vi "Rack-Config.vi"(8 "error in (no error)":errorcluster, 11 "Options":T1={"Input polling period (ms)"=2, "Logfile folder"=path "C:/Users/SiapasLab/Desktop/git/wheatley/test_log.txt"}) -> (0 "error out":errorcluster, 3 "Configuration":T2={"DigitalInput"={"Lines"=["6289/port1/line0", "6289/port1/line1", "6289/port1/line2", "6289/port1/line3", "6289/port1/line4", "6289/port1/line5", "6289/port1/line6", "6289/port1/line7"], "Refresh period (ms)"=0}, "DigitalOutput"={"Output Lines"=["6289/port0/line1", "6289/port0/line2", "6289/port0/line3", "6289/port0/line4", "6289/port0/line5", "6289/port0/line6", "6289/port0/line7"], "DO timestamp lines"=["6289/port0/line1", "6289/port0/line2", "6289/port0/line3", "6289/port0/line4", "6289/port0/line5", "6289/port0/line6", "6289/port0/line7"], "Timestamp lines"=[]}, "FileOutput"={"Logfile path"=path ""}, "AnalogOutput"={"Output Lines"=["6289/port0/line1", "6289/port0/line2", "6289/port0/line3", "6289/port0/line4", "6289/port0/line5", "6289/port0/line6", "6289/port0/line7"], "AO timestamp lines"=["6289/port0/line1", "6289/port0/line2", "6289/port0/line3", "6289/port0/line4", "6289/port0/line5", "6289/port0/line6", "6289/port0/line7"]}, "DataSocketOutput"={"DataSocket URL"=""}})   [LabVIEW 2015]
doc: "Creates an appropriate configuration cluster for use in Rack-Start.vi\n\nOptions are specified in this VI's front panel, but can be overwritten by the calling VI (just use bundle by name).\n\nCall this after all devices are initialized, as it uses the port reservation system to find which lines to assign to each port driver."
uses:
  Typedefs/Rack driver configuration cluster.ctl
  Port drivers/DigitalInput-Configuration.ctl
  Port drivers/DigitalOutput-Configuration.ctl
  Port drivers/FileOutput-Configuration.ctl
  Port drivers/AnalogOutput-Configuration.ctl
  Port drivers/DataSocketOutput-Configuration.ctl
panel:
  # "Timestamp lines must be on an M-Series card (i.e. NOT the 6509)"
  # "Timestamp lines must be on same device as its corresponding DO line"
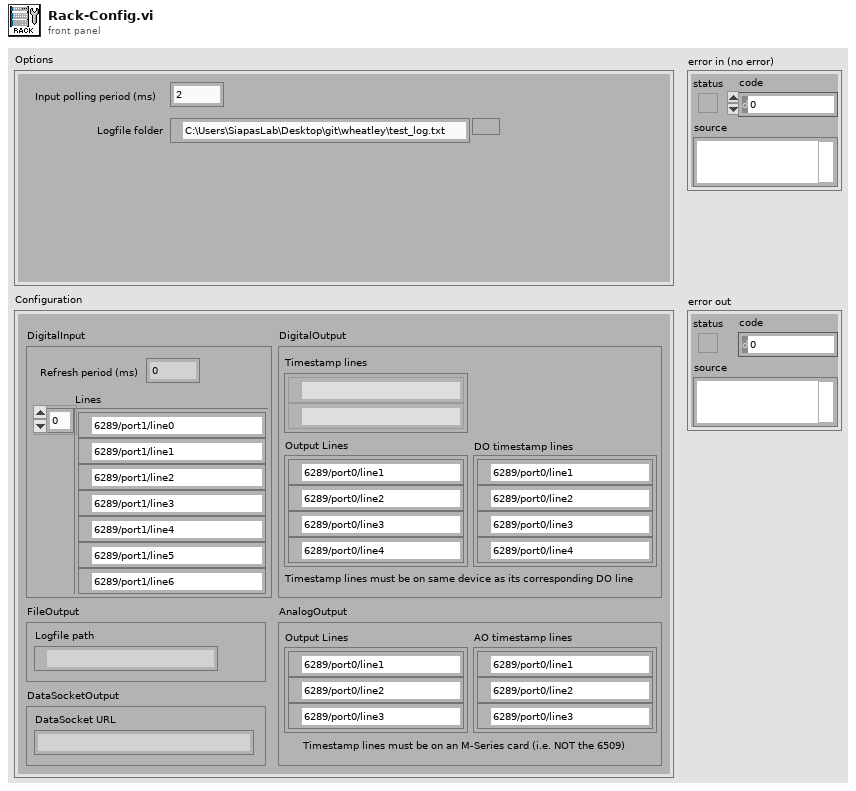
[diagram p1: front panel]
types:
  T1 = cluster{"Input polling period (ms)":u32, "Logfile folder":path}
  T2 = typedef "Rack driver configuration cluster.ctl" = cluster{"DigitalInput":T3, "DigitalOutput":T4, "FileOutput":T5, "AnalogOutput":T6, "DataSocketOutput":T7}
  T3 = typedef "DigitalInput-Configuration.ctl" = cluster{"Lines":tag[], "Refresh period (ms)":u32}
  T4 = typedef "DigitalOutput-Configuration.ctl" = cluster{"Output Lines":tag[], "DO timestamp lines":tag[], "Timestamp lines":tag[]}
  T5 = typedef "FileOutput-Configuration.ctl" = cluster{"Logfile path":path}
  T6 = typedef "AnalogOutput-Configuration.ctl" = cluster{"Output Lines":tag[], "AO timestamp lines":tag[]}
  T7 = typedef "DataSocketOutput-Configuration.ctl" = cluster{"DataSocket URL":string}
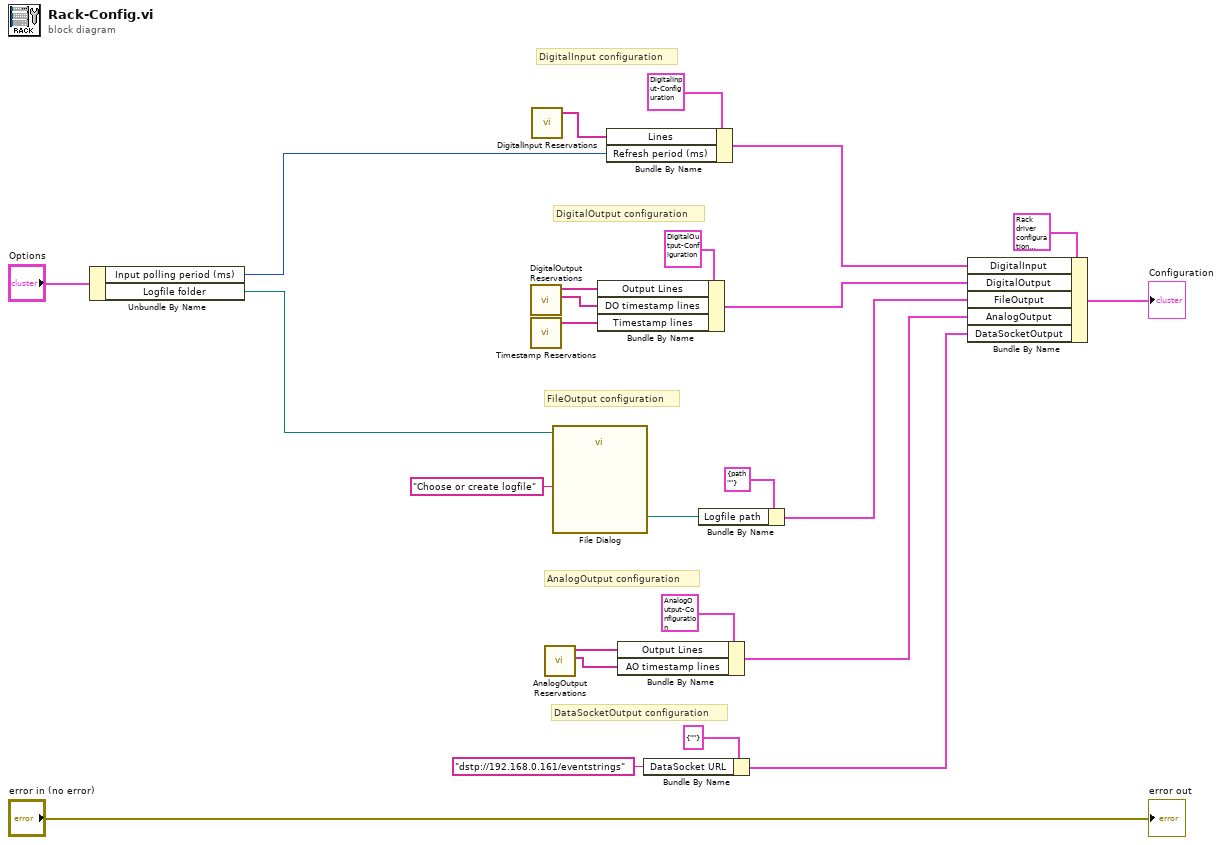
[diagram p0: block diagram]
diagram:
  # "DataSocketOutput configuration"
  # "AnalogOutput configuration"
  # "FileOutput configuration"
  # "DigitalOutput configuration"
  # "DigitalInput configuration"
  n1 = Unbundle By Name("Options") -> ("Input polling period (ms)"=w20:u32, "Logfile folder"=w14:path)
  n2 = call "DigitalOutput Reservations.vi"() -> ("DO timestamp lines"=w9:tag[], "DigitalOutput lines"=w17:tag[])  [unwired: 4 in, 2 out]
  n3 = call "Timestamp Reservations.vi"() -> ("DigitalOutput lines"=w8:tag[])  [unwired: 3 in, 2 out]
  n4 = call "DigitalInput Reservations.vi"() -> ("DigitalInput lines"=w19:tag[])  [unwired: 3 in, 2 out]
  n5 = call "AnalogOutput Reservations.vi"() -> ("AO timestamp lines"=w4:tag[], "AnalogOutput lines"=w5:tag[])  [unwired: 4 in, 2 out]
  n6 = call "File Dialog"("start path"=w14, "prompt"="Choose or create logfile") -> ("selected path"=w10:path)  [unwired: 10 in, 3 out]
  n7 = Bundle By Name(cluster=T4 {"Output Lines"=["6289/port0/line3", "6289/port0/line4", "6289/port0/line5", "6289/port0/line6", "6289/port0/line7"], "DO timestamp lines"=[], "Timestamp lines"=[]} ("DigitalOutput"), "Output Lines"=w17, "DO timestamp lines"=w9, "Timestamp lines"=w8) -> (w15:T4)
  n8 = Bundle By Name(cluster=T3 {"Lines"=["6289/port1/line0", "6289/port1/line1", "6289/port1/line2", "6289/port1/line3", "6289/port1/line4", "6289/port1/line5", "6289/port1/line6", "6289/port1/line7"], "Refresh period (ms)"=0} ("DigitalInput"), "Lines"=w19, "Refresh period (ms)"=w20) -> (w16:T3)
  n9 = Bundle By Name(cluster=T6 {"Output Lines"=["6289/port0/line1", "6289/port0/line2", "6289/port0/line3", "6289/port0/line4", "6289/port0/line5", "6289/port0/line6", "6289/port0/line7"], "AO timestamp lines"=["6289/port0/line1", "6289/port0/line2", "6289/port0/line3", "6289/port0/line4", "6289/port0/line5", "6289/port0/line6", "6289/port0/line7"]} ("AnalogOutput"), "Output Lines"=w5, "AO timestamp lines"=w4) -> (w6:T6)
  n10 = Bundle By Name(cluster=T7 {"DataSocket URL"=""} ("DataSocketOutput"), "DataSocket URL"="dstp://192.168.0.161/eventstrings") -> (w2:T7)
  n11 = Bundle By Name(cluster=T5 {"Logfile path"=path ""} ("FileOutput"), "Logfile path"=w10) -> (w11:T5)
  n12 = Bundle By Name(cluster=T2 {"DigitalInput"={"Lines"=["", "6289/port1/line1", "6289/port1/line2", "6289/port1/line3", "6289/port1/line4", "6289/port1/line5", "6289/port1/line6", "6289/port1/line7"], "Refresh period (ms)"=0}, "DigitalOutput"={"Output Lines"=["", "6289/port0/line2", "6289/port0/line3", "6289/port0/line4", "6289/port0/line5", "6289/port0/line6", "6289/port0/line7"], "DO timestamp lines"=[], "Timestamp lines"=[]}, "FileOutput"={"Logfile path"=path ""}, "AnalogOutput"={"Output Lines"=[], "AO timestamp lines"=[]}, "DataSocketOutput"={"DataSocket URL"=""}} ("Configuration"), "DigitalInput"=w16, "DigitalOutput"=w15, "FileOutput"=w11, "AnalogOutput"=w6, "DataSocketOutput"=w2) -> (→"Configuration":T2)
  "error out" <- "error in (no error)"
